vi "Compare Images.vi"(7 "Compare Method":T2=enum."Peak Signal-to-Noise Ratio", 8 "error in (no error)":errorcluster, 10 "Actual Image":T1, 11 "Expected Image":T1) -> (0 "error out":errorcluster, 3 "Value":dbl)   [LabVIEW 2020, in "MacroAssert.lvlib" / "Image Assertion.lvclass"]
uses:
  Image Assertion.lvclass
  Compare Method.ctl
  <vilib>/picture/picture.llb/imagedata.ctl
  <vilib>/Utility/error.llb/Error Cluster From Error Code.vi
  SubVIs/Custom Errors/Custom Errors.lvlib
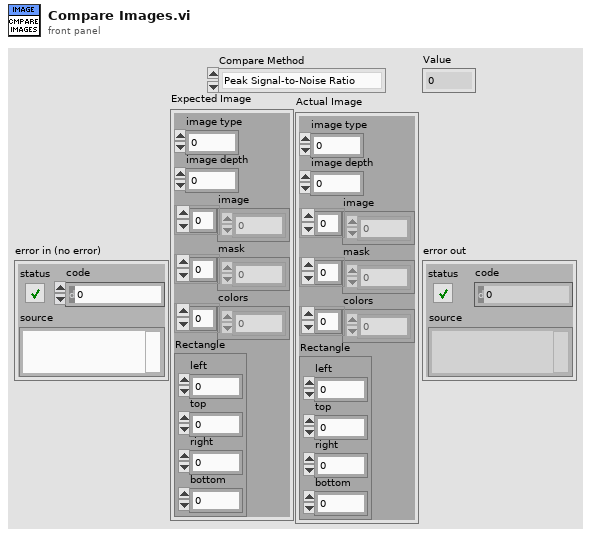
[diagram p1: front panel]
types:
  T1 = typedef "imagedata.ctl" = cluster{"image type":i32, "image depth":i32, "image":u8[], "mask":u8[], "colors":u32[], "Rectangle":cluster{"left":i16, "top":i16, "right":i16, "bottom":i16}}
  T2 = typedef "MacroAssert.lvlib/Image Assertion.lvclass/Compare Method.ctl" = enum16{"Mean Squared Error", "Peak Signal-to-Noise Ratio"}
  T3 = cluster{"left":i16, "top":i16, "right":i16, "bottom":i16}
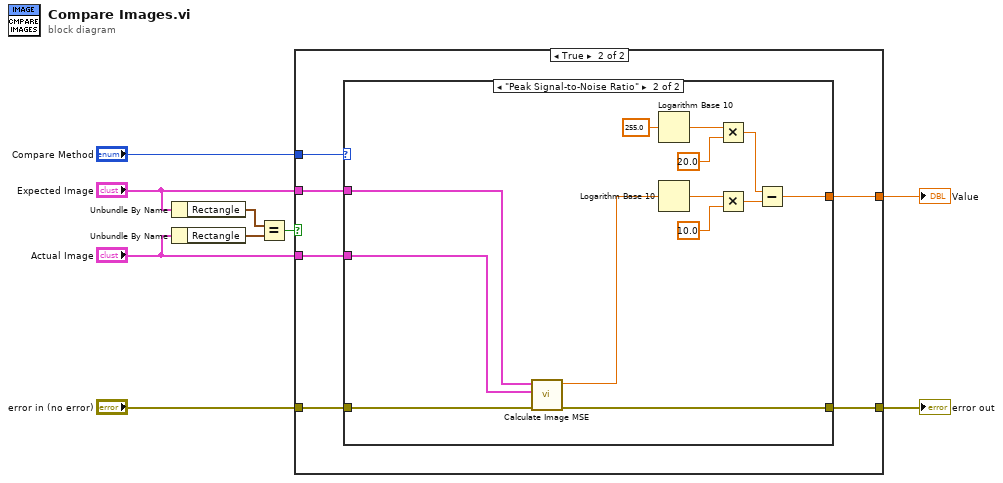
[diagram p0: block diagram]
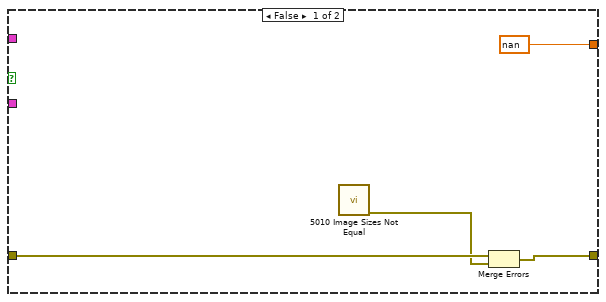
[diagram p2: hidden frame]
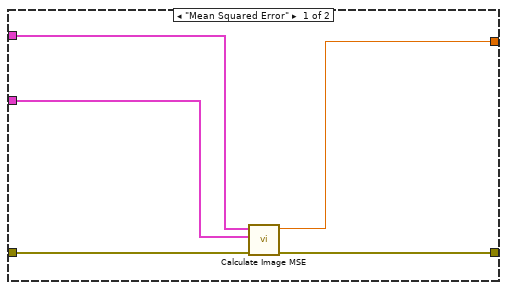
[diagram p3: hidden frame]
diagram:
  n1 = Unbundle By Name("Expected Image") -> ("Rectangle"=w5:T3)
  n2 = Unbundle By Name("Actual Image") -> ("Rectangle"=w4:T3)
  n3 = Equal?(x=w5, y=w4) -> (x = y?=w1:bool)
  n4 = case shown="True" w1 {
    tunnel: [nan w19] -> w9
    tunnel: "Compare Method" -> [_ w18]
    tunnel: "error in (no error)" -> [w12 w17]
    tunnel: [w10 w16] -> w6
    tunnel: "Actual Image" -> [_ w15]
    tunnel: "Expected Image" -> [_ w14]
    frame False {
      n5 = call "5010 Image Sizes Not Equal.vi"() -> ("error out"=w11:errorcluster)  [unwired: 11 in]
      n6 = Merge Errors(w12, w11) -> (w10:errorcluster)
    }
    frame True {
      n7 = case shown="\"Peak Signal-to-Noise Ratio\"" w18 {
        tunnel: [w20 w32] -> w19
        tunnel: w17 -> [w24 w29]
        tunnel: [w23 w26] -> w16
        tunnel: w15 -> [w21 w27]
        tunnel: w14 -> [w22 w28]
        frame "Mean Squared Error" {
          n8 = call "Calculate Image MSE.vi"("error in (no error)"=w24, "Actual Image"=w21, "Expected Image"=w22) -> ("error out"=w23:errorcluster, "MSE"=w20:dbl)  [unwired: 7 in]
        }
        frame "Peak Signal-to-Noise Ratio" {
          n9 = call "Calculate Image MSE.vi"("error in (no error)"=w29, "Actual Image"=w27, "Expected Image"=w28) -> ("error out"=w26:errorcluster, "MSE"=w25:dbl)  [unwired: 7 in]
          n10 = Logarithm Base 10(1:255.0 ("x")) -> (0:w34:dbl)
          n11 = Logarithm Base 10(1:w25) -> (0:w37:dbl)
          n12 = Multiply(x=w34, y=20.0) -> (x*y=w30:dbl)
          n13 = Multiply(x=w37, y=10.0) -> (x*y=w31:dbl)
          n14 = Subtract(x=w30, y=w31) -> (x-y=w32:dbl)
        }
      }
    }
  }
  "Value" <- w9
  "error out" <- w6
